vi "Create Digital Pattern.vi"(6 "Timeout (10000 ms)":u32=10000, 8 "error in (no error)":errorcluster, 9 "Digital Pattern Data":u16[](array[numeric]), 10 "Digital Pattern Name (\"PAT1\")":string="PAT1", 11 "VISA resource name":refnum<visa-resource-name>) -> (0 "error out":errorcluster, 3 "VISA resource name out":refnum<visa-resource-name>)   [LabVIEW 2017, in "Keithley 3390.lvlib"]
doc: "Creates and saves an arbitrary (user-defined) digital pattern in non-volatile memory."
uses:
  Keithley 3390.lvlib
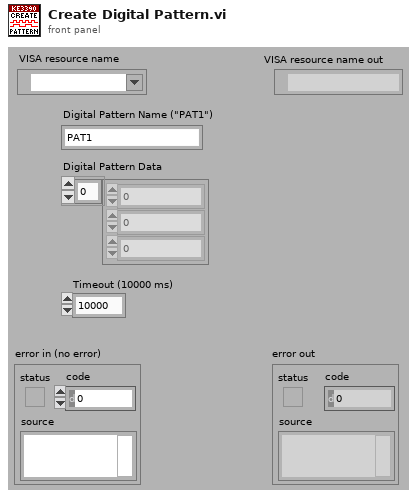
[diagram p1: front panel]
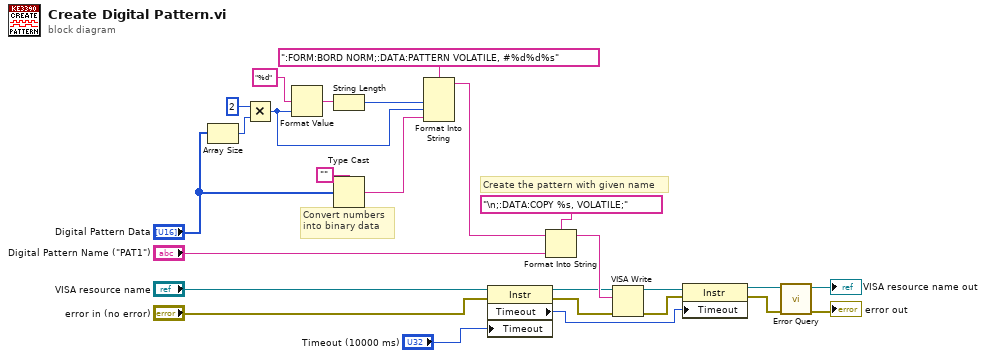
[diagram p0: block diagram]
diagram:
  # "Convert numbers\ninto binary data"
  # "Create the pattern with given name"
  n1 = Array Size(array="Digital Pattern Data") -> (size(s)=w5:i32)
  n2 = Multiply(x=2, y=w5) -> (x*y=w17:i32)
  n3 = Format Value(format string="%d", value (0)=w17) -> (output string=w8:string)  [unwired: 1 in]
  n4 = String Length(string=w8) -> (length=w16:i32)
  n5 = Type Cast(type="", x="Digital Pattern Data") -> (*(type *) &x=w18:string)
  n6 = Format Into String(format string=":FORM:BORD NORM;:DATA:PATTERN VOLATILE, #%d%d%s" ("string"), w16, w17, w18) -> (resulting string=w20:string)  [unwired: 2 in, 1 out]
  n7 = property class="Instr"(reference="VISA resource name", error in="error in (no error)", "Timeout"="Timeout (10000 ms)") -> (reference out=w10:refnum<visa-resource-name>, error out=w9:errorcluster, "Timeout"=w13:u32)
  n8 = Format Into String(format string="\n;:DATA:COPY %s, VOLATILE;", initial string=w20, "Digital Pattern Name (\"PAT1\")") -> (resulting string=w22:string)  [unwired: 1 in, 1 out]
  n9 = VISA Write(VISA resource name=w10, write buffer=w22, error in (no error)=w9) -> (VISA resource name out=w11:refnum<visa-resource-name>, error out=w12:errorcluster)  [unwired: 1 out]
  n10 = property class="Instr"(reference=w11, error in=w12, "Timeout"=w13) -> (reference out=w24:refnum<visa-resource-name>, error out=w25:errorcluster)
  n11 = call "Error Query.vi"("error in (no error)"=w25, "VISA resource name"=w24) -> ("error out"=→"error out":errorcluster, "VISA resource name out"=→"VISA resource name out":refnum<visa-resource-name>)  [unwired: 6 in, 2 out]
